vi "Convert Parse to Command Arquements.vi"(8 "error in (no error)":errorcluster, 11 "Address Parsed Tree":T1) -> (0 "error out":errorcluster, 2 "Type":string, 3 "Address":string)   [LabVIEW 2013, in "J1939 Addon Shared.lvlib"]
uses:
  J1939 Addon Shared.lvlib
  Types/Address Parse Tree Cluster.ctl
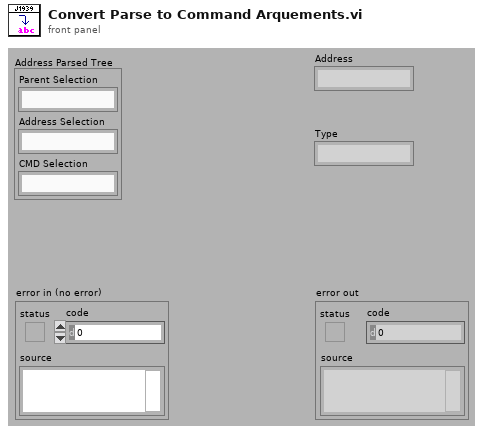
[diagram p1: front panel]
types:
  T1 = typedef "J1939 Addon Shared.lvlib/Address Parse Tree Cluster.ctl" = cluster{"Parent Selection":string, "Address Selection":string, "CMD Selection":string}
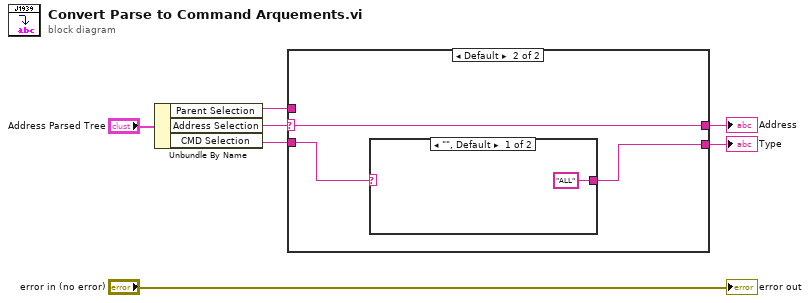
[diagram p0: block diagram]
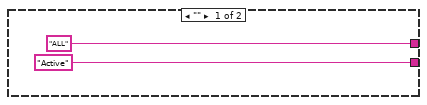
[diagram p2: hidden frame]
diagram:
  n1 = Unbundle By Name("Address Parsed Tree") -> ("Parent Selection"=w5:string, "Address Selection"=w6:string, "CMD Selection"=w4:string)
  n2 = case shown="Default" w6 {
    selector: w6 -> [_ w12]
    tunnel: w5 -> [_ _]
    tunnel: ["ALL" w12] -> w3
    tunnel: w4 -> [_ w11]
    tunnel: ["Active" w10] -> w2
    frame "" {
    }
    frame Default {
      n3 = case shown="\"\", Default" w11 {
        selector: w11 -> [_ w14]
        tunnel: ["ALL" w14] -> w10
        frame "", Default {
        }
        frame "Active", "Previous" {
        }
      }
    }
  }
  "Address" <- w3
  "Type" <- w2
  "error out" <- "error in (no error)"
